vi "GetCorrectPositions.vi"(9 "Field Size in":T1, 11 "Posição dos defensores":dbl[][](array[numeric]) format="%#_13g") -> (3 "Posição dos defensores correta":dbl[][](array[numeric]) format="%#_13g")   [LabVIEW 2017]
uses:
  Core/Field Size.ctl
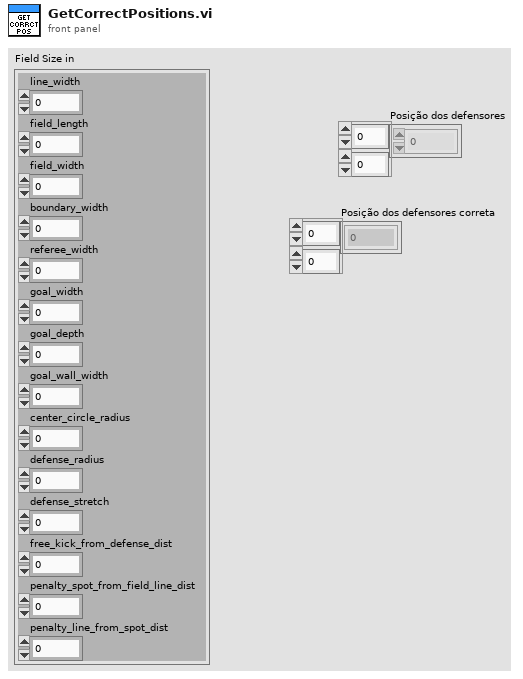
[diagram p1: front panel]
types:
  T1 = typedef "Field Size.ctl" = cluster{"line_width":u32, "field_length":u32, "field_width":u32, "boundary_width":u32, "referee_width":u32, "goal_width":u32, "goal_depth":u32, "goal_wall_width":u32, "center_circle_radius":u32, "defense_radius":u32, "defense_stretch":u32, "free_kick_from_defense_dist":u32, "penalty_spot_from_field_line_dist":u32, "penalty_line_from_spot_dist":u32}
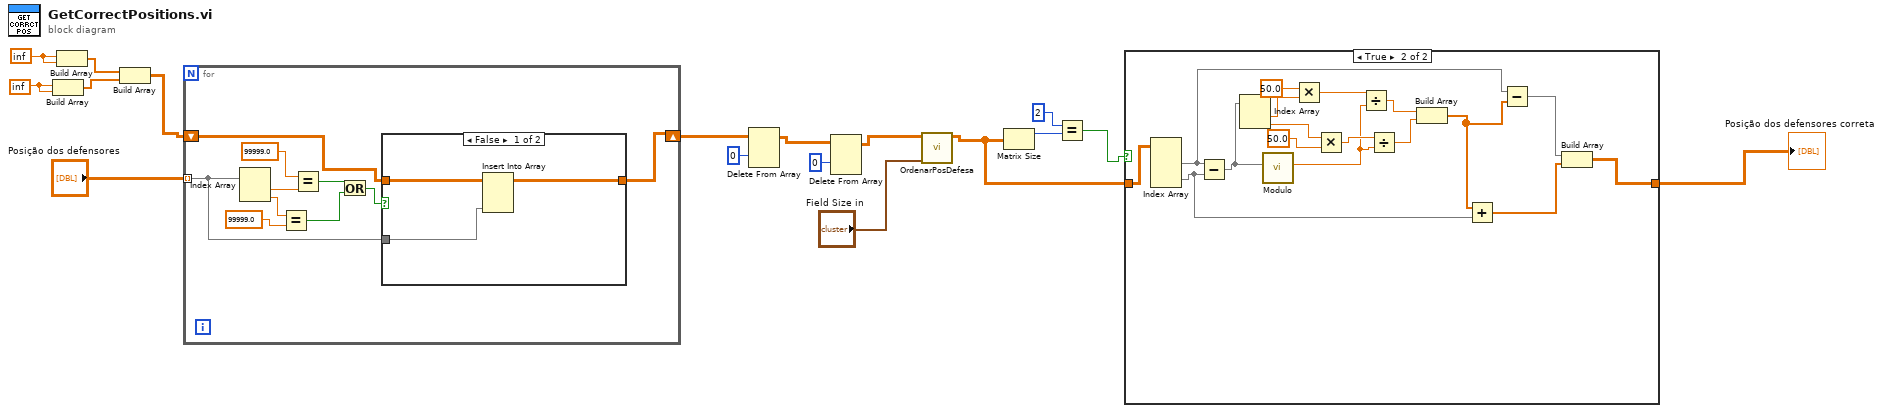
[diagram p0: block diagram]
diagram:
  w15 = inf
  w16 = inf
  n1 = Build Array(w15, w15) -> (w13:dbl[])
  n2 = Build Array(w16, w16) -> (w14:dbl[])
  n3 = Build Array(w14, w13) -> (w10:dbl[][])
  n4 = for {
    tunnel: "Posição dos defensores" -> [w20] mode=indexing
    shift-right: [w19] -> w12
    shift-left: w10 -> [w18]
    n5 = Index Array(array=w20) -> (element #1=w27:dbl, element #2=w24:dbl)  [unwired: 2 in]
    n6 = Equal?(x=w24, y=99999.0 ("x")) -> (x = y?=w22:bool)
    n7 = Equal?(x=99999.0, y=w27) -> (x = y?=w23:bool)
    n8 = Or(x=w23, y=w22) -> (x .or. y?=w21:bool)
    n9 = case shown="False" w21 {
      tunnel: w20 -> [w30 _]
      tunnel: [w29 w31] -> w19
      tunnel: w18 -> [w28 w31]
      frame False {
        n10 = Insert Into Array(array=w28, new element=w30) -> (w29:dbl[][])  [unwired: 2 in]
      }
      frame True {
      }
    }
  }
  n11 = Delete From Array(array=w12, index (row)=0) -> (array with subset deleted=w8:dbl[][])  [unwired: 2 in, 1 out]
  n12 = Delete From Array(array=w8, index (row)=0) -> (array with subset deleted=w7:dbl[][])  [unwired: 2 in, 1 out]
  n13 = call "OrdenarPosDefesa.vi"("geometry"="Field Size in", "Posições da defesa"=w7) -> ("Posições ordenadas"=w1:dbl[][])  [unwired: 9 in]
  n14 = Matrix Size(0:w1) -> (1:w5:i32)  [unwired: 1 out]
  n15 = Equal?(x=2, y=w5) -> (x = y?=w3:bool)
  n16 = case shown="True" w3 {
    tunnel: [w32 w33] -> w2
    tunnel: w1 -> [w32 w49]
    frame False {
    }
    frame True {
      n17 = Index Array(array=w49) -> (element #1=w36:dbl[], element #2=w38:dbl[])  [unwired: 4 in]
      n18 = Subtract(x=w36, y=w38) -> (x-y=w48:dbl[])
      n19 = Index Array(array=w48) -> (element #1=w47:dbl, element #2=w44:dbl)  [unwired: 2 in]
      n20 = call "Modulo.vi"("2D vector"=w48) -> ("Modulo"=w41:dbl)  [unwired: 10 in]
      n21 = Multiply(x=50.0, y=w47) -> (x*y=w43:dbl)
      n22 = Multiply(x=w44, y=50.0 ("x")) -> (x*y=w42:dbl)
      n23 = Divide(x=w43, y=w41) -> (x/y=w40:dbl)
      n24 = Divide(x=w42, y=w41) -> (x/y=w39:dbl)
      n25 = Build Array(w40, w39) -> (w37:dbl[])
      n26 = Add(x=w37, y=w38) -> (x+y=w34:dbl[])
      n27 = Subtract(x=w36, y=w37) -> (x-y=w35:dbl[])
      n28 = Build Array(w35, w34) -> (w33:dbl[][])
    }
  }
  "Posição dos defensores correta" <- w2
